vi "Autonomous.vi"() -> (2 "Switch to teleop":bool=TRUE, 3 "output cluster":T1={"Team Number"="3492", "Autonomous Comments"="", "Autonomous?"="Yes", "Did they pick up more discs?"="No", "1 Point"=0.0, "2 Points"=0.0, "3 Points"=0.0})   [LabVIEW 2014]
panel:
  in  "Did they pick up more discs?":string(combo)="No"
  in  "Autonomous?":string(combo)="No"
  in  "SWITCH TO TELEOP":bool
  in  "Team Number":string
  in  "Autonomous Comments":string
  in  "3 Points":dbl
  in  "1 Point":dbl
  in  "2 Points":dbl
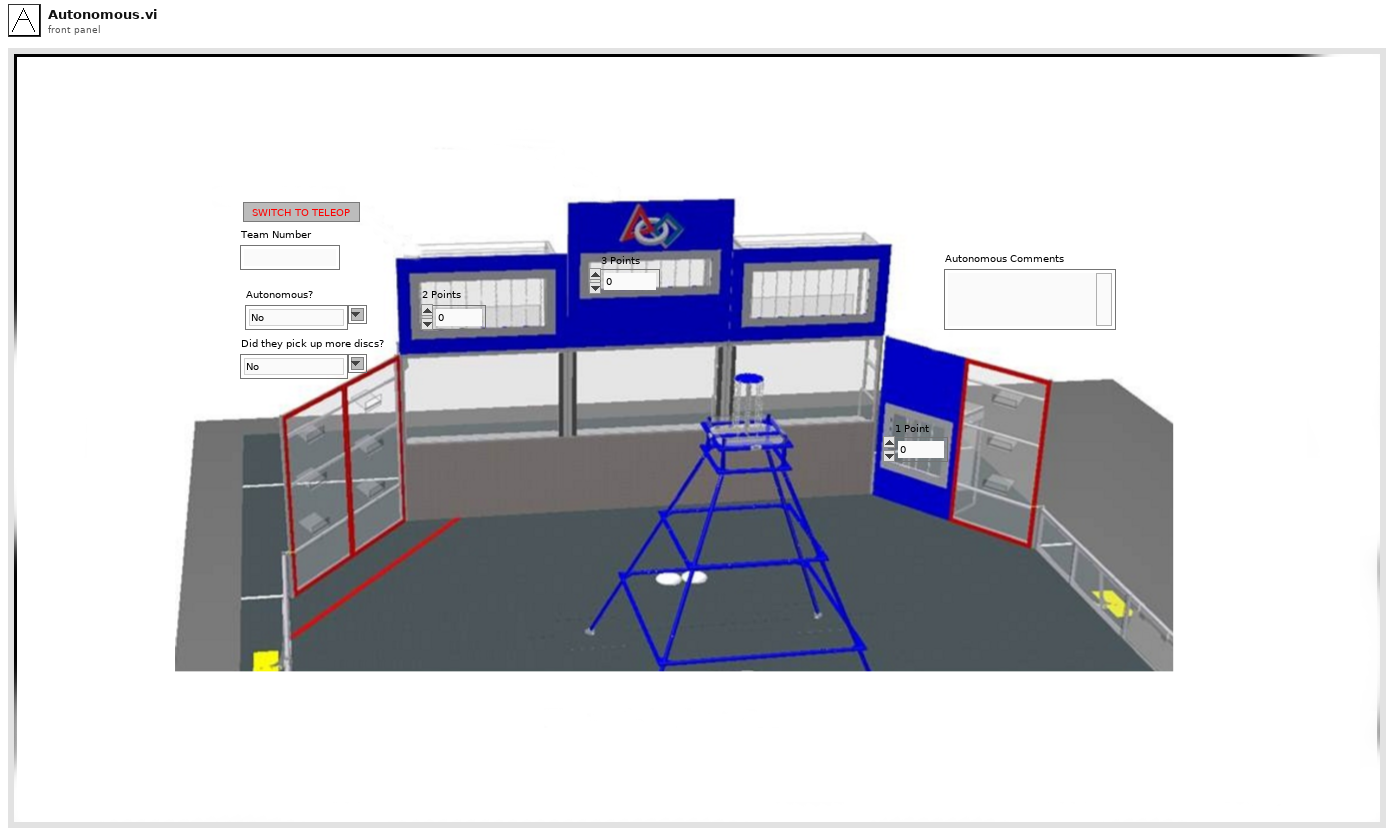
[diagram p1: front panel]
types:
  T1 = cluster{"Team Number":string, "Autonomous Comments":string, "Autonomous?":string, "Did they pick up more discs?":string, "1 Point":dbl, "2 Points":dbl, "3 Points":dbl}
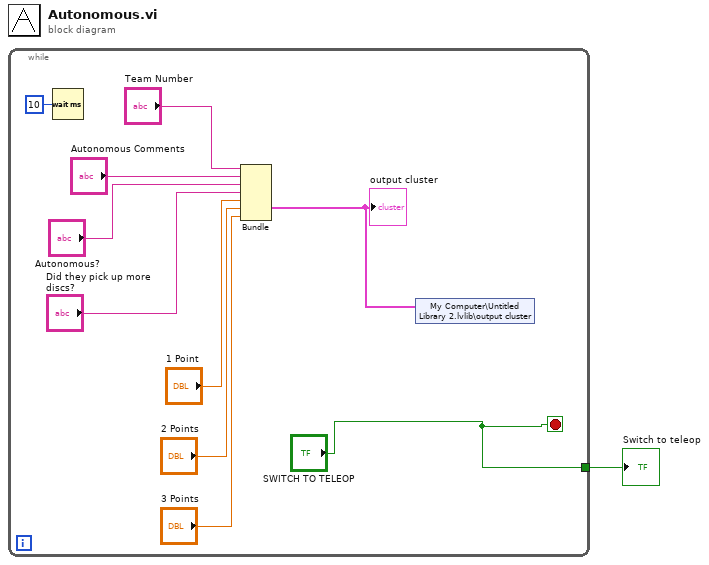
[diagram p0: block diagram]
diagram:
  n1 = while {
    tunnel: ["SWITCH TO TELEOP"] -> w1
    stop <- "SWITCH TO TELEOP" stop-if-true
    n2 = Wait (ms)(milliseconds to wait=u32 10) -> ()  [unwired: 1 out]
    n3 = Bundle("Team Number"="Team Number", "Autonomous Comments"="Autonomous Comments", "Autonomous?"="Autonomous?", "Did they pick up more discs?"="Did they pick up more discs?", "1 Point"="1 Point", "2 Points"="2 Points", "3 Points"="3 Points") -> (w2:T1)  [unwired: 1 in]
    "output cluster" <- w2
    n4 = shared-variable "My Computer\\Untitled Library 2.lvlib\\output cluster"(w2) -> ()  [unwired: 1 in, 1 out]
  }
  "Switch to teleop" <- w1
